vi "Vision Main.vi"(10 "Frame Buffer":T1, 11 "Camera Image":T1(plugin-control)) -> (2 "Chosen Target Angle":dbl, 3 "Sorted Targets":T2(array[cluster]))   [LabVIEW 2012]
uses:
  <vilib>/vision/Image Controls.llb/IMAQ Image.ctl
panel:
  out "Particle Reports (Pixels)":T3(array[cluster]) {"Orientation" format="%.2f"; "Dimensions"."Height" format="%.2f"; "Dimensions"."Width" format="%.2f"; "Center of Mass"."Y" format="%.2f"; "Center of Mass"."X" format="%.2f"; "Bounding Rect"."Bottom" format="%.2f"; "Bounding Rect"."Right" format="%.2f"; "Bounding Rect"."Top" format="%.2f"; "Bounding Rect"."Left" format="%.2f"; "Number of Holes" format="%.2f"; "Area" format="%.2f"}
  out "Number of Particles":i32
  out "Processed Image":T1(plugin-control)
  out "Cropped Image":T1(plugin-control)
  # "Camera Image"
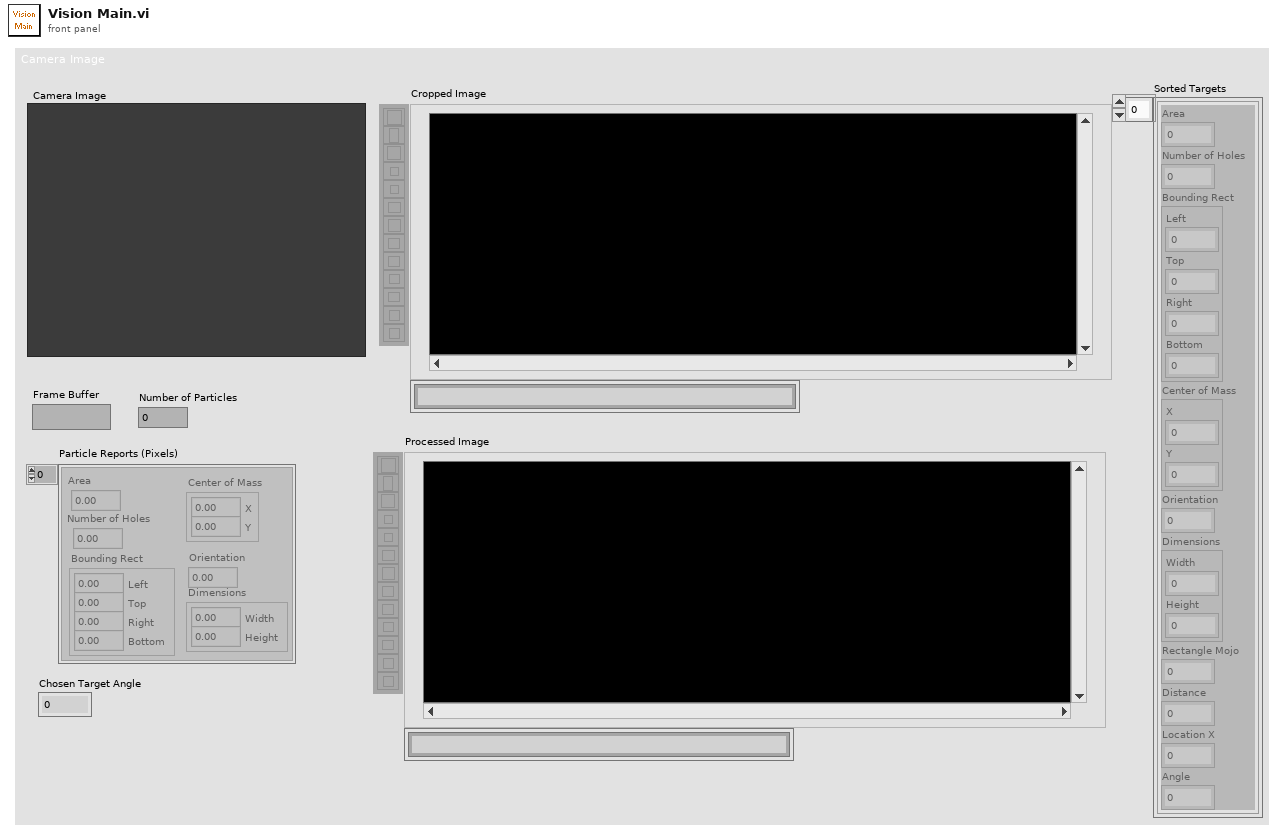
[diagram p1: front panel]
types:
  T1 = typedef "IMAQ Image.ctl" = refnum<image>
  T2 = cluster{"Area":dbl, "Number of Holes":dbl, "Bounding Rect":cluster{"Left":dbl, "Top":dbl, "Right":dbl, "Bottom":dbl}, "Center of Mass":cluster{"X":dbl, "Y":dbl}, "Orientation":dbl, "Dimensions":cluster{"Width":dbl, "Height":dbl}, "Rectangle Mojo":dbl, "Distance":dbl, "Location X":dbl, "Angle":dbl}[]
  T3 = cluster{"Area":dbl, "Number of Holes":dbl, "Bounding Rect":cluster{"Left":dbl, "Top":dbl, "Right":dbl, "Bottom":dbl}, "Center of Mass":cluster{"X":dbl, "Y":dbl}, "Orientation":dbl, "Dimensions":cluster{"Width":dbl, "Height":dbl}}[]
  T4 = typedef "Image Type" = u32
  T5 = cluster{"Area":dbl, "Number of Holes":dbl, "Bounding Rect":cluster{"Left":dbl, "Top":dbl, "Right":dbl, "Bottom":dbl}, "Center of Mass":cluster{"X":dbl, "Y":dbl}, "Orientation":dbl, "Dimensions":cluster{"Width":dbl, "Height":dbl}, "Rectangle Mojo":dbl, "Distance":dbl, "Location X":dbl, "Angle":dbl}
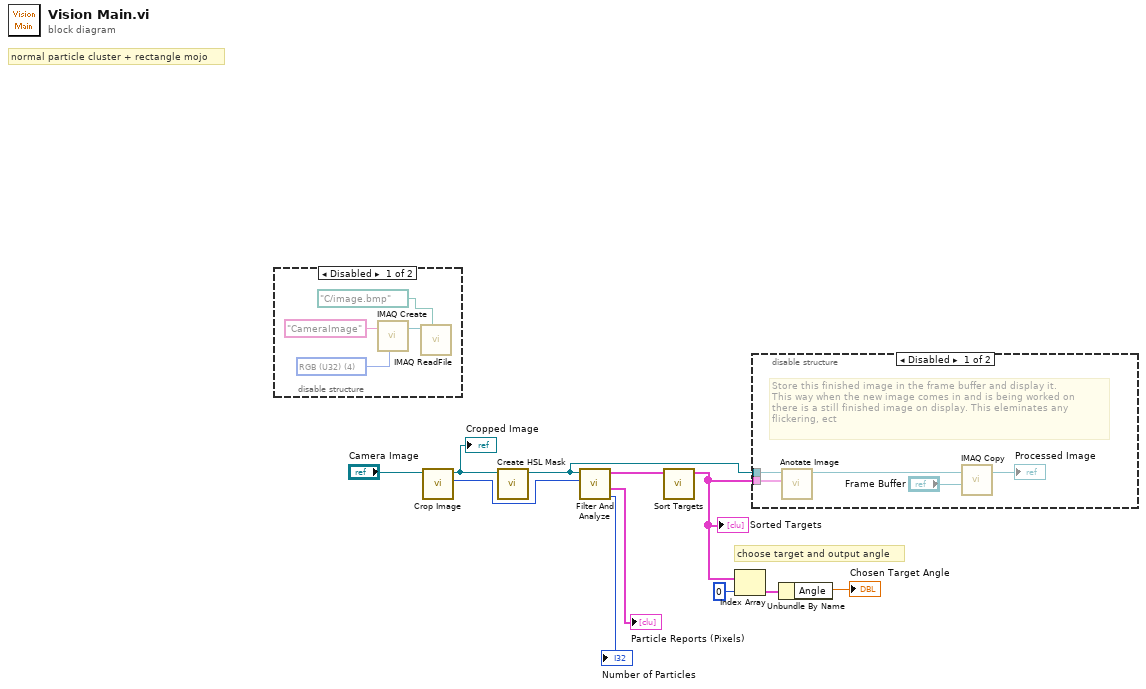
[diagram p0: block diagram]
diagram:
  # "choose target and output angle"
  # "normal particle cluster + rectangle mojo"
  n1 = disable-structure shown="Disabled" {
    frame Disabled {
      w13 = T4 4 items=["Grayscale (U8)", "Grayscale (I16)", "Grayscale (SGL)", "Complex (CSG)", "RGB (U32)", "HSL (U32)", "RGB (U64)", "Grayscale (U16)"] ("Image Type")
      n2 = call "IMAQ Create"("Image Name"="CameraImage", "Image Type"=w13) -> ("New Image"=w16:T1)  [unwired: 3 in, 1 out]
      n3 = call "IMAQ ReadFile"("File Path"=path "C:/image.bmp", "Image"=w16) -> ("Image Out"=w12:T1)  [unwired: 5 in, 4 out]
    }
    frame Enabled {
    }
  }
  n4 = call "Crop Image.vi"("Camera Image"="Camera Image") -> ("Y Resolution"=w8:i32, "Cropped Image"=w10:T1)  [unwired: 8 in, 1 out]
  "Cropped Image" <- w10
  n5 = call "Create HSL Mask.vi"("Cropped Image"=w10) -> ("Image Mask"=w9:T1)  [unwired: 10 in]
  n6 = call "Filter And Analyze.vi"("Y Resolution"=w8, "Refnum in"=w9) -> ("Number of Particles"=→"Number of Particles":i32, "Particle Reports (Pixels)"=→"Particle Reports (Pixels)":T3, "Filtered Array"=w7:T2)  [unwired: 7 in]
  n7 = call "Sort Targets.vi"("Filtered Array"=w7) -> ("Sorted Array"=w4:T2)  [unwired: 10 in]
  "Sorted Targets" <- w4
  n8 = Index Array(array=w4, index=0) -> (element=w2:T5)
  n9 = disable-structure shown="Disabled" {
    disable-tunnel: w9 -> [w20 _]
    disable-tunnel: w4 -> [w18 _]
    frame Disabled {
      # "Store this finished image in the frame buffer and display it.\nThis way when the new image comes in and is being worked on\nthere is a still finished image on display. This eleminates any\nflickering, ect"
      n10 = call "Anotate Image.vi"("Sorted Array"=w18, "Image Refnum in"=w20) -> ("Image Refnum out"=w21:T1)  [unwired: 9 in]
      n11 = call "IMAQ Copy"("Image Dst"="Frame Buffer", "Image Src"=w21) -> ("Image Dst Out"=→"Processed Image":T1)  [unwired: 4 in, 1 out]
    }
    frame Enabled {
      # "only enable this for debuging to see the processed image\nnormally we never need to see this"
    }
  }
  n12 = Unbundle By Name(w2) -> ("Angle"=→"Chosen Target Angle":dbl)
